vi "temp.vi"(8 "error in (no error)":errorcluster, 10 "TestCase out 2":refnum<class "TestCase.lvclass">, 11 "WasRun in":refnum<class "WasRun.lvclass">) -> (0 "error out":errorcluster, 3 "WasRun out":refnum<class "WasRun.lvclass">)   [LabVIEW 2013, in "WasRun.lvclass"]
uses:
  WasRun.lvclass
  <vilib>/addons/_JKI Toolkits/VI Tester/TestCase.llb/TestCase.lvclass
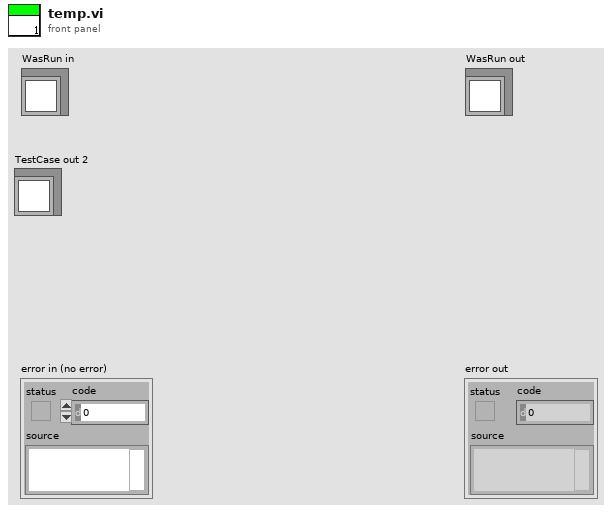
[diagram p1: front panel]
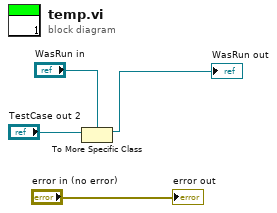
[diagram p0: block diagram]
diagram:
  n1 = To More Specific Class(target class="WasRun in", reference="TestCase out 2") -> (specific class reference=→"WasRun out":refnum<class "WasRun.lvclass">)  [unwired: 1 in, 1 out]
  "error out" <- "error in (no error)"
